vi "Measure_V_1.vi"(8 "errin":errorcluster, 11 "multi":refnum<visa-resource-name>) -> (0 "errout":errorcluster, 3 "Measurement":dbl)   [LabVIEW 2020]
uses:
  <vilib>/Instr/_visa.llb/VISA Open Access Mode.ctl
  <instrlib>/Agilent 3446X Series/Public/Data/Read (Single Point).vi
  <instrlib>/Agilent 3446X Series/Agilent 3446X Series.lvlib
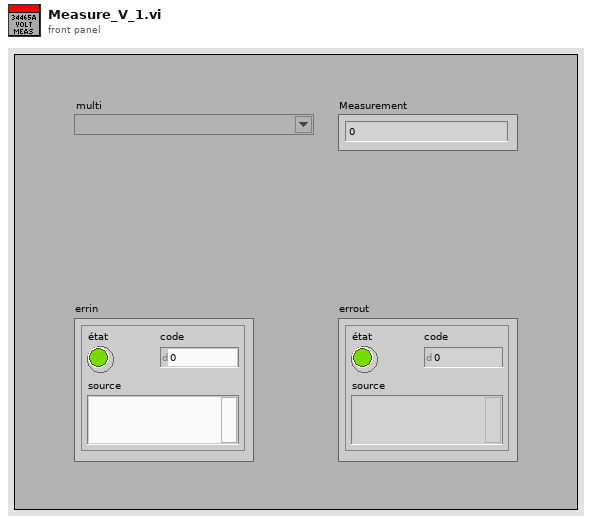
[diagram p1: front panel]
types:
  T1 = typedef "VISA Open Access Mode.ctl" = u32
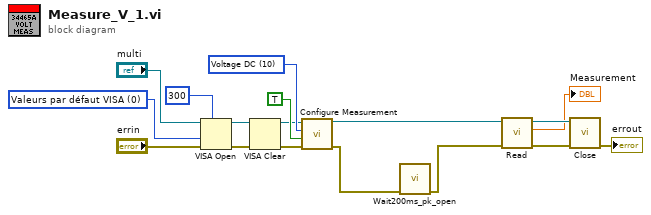
[diagram p0: block diagram]
diagram:
  w16 = 10 items=["Continuity", "Current AC", "Current DC", "Diode", "Frequency", "Resistance 4-wire", "Period", "Resistance 2-wire", "Temperature", "Voltage AC", "Voltage DC", "Voltage DC Ratio", "Capacitance"] ("fonction")
  w7 = T1 0 items=["Valeurs par défaut VISA"=0, "Verrouillage exclusif"=1, "Charger les paramètres configurés"=4] ("Access Mode")
  n1 = VISA Open(timeout (0)=u32 300 ("Timeout de VISA Open (0)"), access mode=w7, error in (no error)="errin", VISA resource name="multi") -> (VISA resource name=w5:refnum<visa-resource-name>, error out=w6:errorcluster)  [unwired: 1 out]
  n2 = VISA Clear(VISA resource name=w5, error in (no error)=w6) -> (VISA resource name out=w10:refnum<visa-resource-name>, error out=w11:errorcluster)
  n3 = call <instrlib>:"Configure Measurement.vi"("error in (no error)"=w11, "Auto Range (T: Enable)"=TRUE, "Measurement Function (10: Voltage DC)"=w16, "VISA resource name"=w10) -> ("error out"=w2:errorcluster, "VISA resource name out"=w12:refnum<visa-resource-name>)  [unwired: 6 in]
  n4 = call "Wait200ms_pk_open.vi"("errin"=w2) -> ("errout"=w1:errorcluster)  [unwired: 10 in]
  n5 = call-poly <instrlib>:"Read.vi"("error in (no error)"=w1, "VISA resource name"=w12) -> ("error out"=w14:errorcluster, "Measurement"=→"Measurement":dbl, "VISA resource name out"=w15:refnum<visa-resource-name>)  [unwired: 7 in]
  n6 = call <instrlib>:"Close.vi"("error in (no error)"=w14, "VISA resource name"=w15) -> ("error out"=→"errout":errorcluster)  [unwired: 9 in]
